vi "Read Variable_Values.vi"(8 "error in (no error)":errorcluster, 11 "muExpr in":refnum<class "mupExpr.lvclass">) -> (0 "error out":errorcluster, 2 "varValues":dbl[](array[numeric]), 3 "muExpr out":refnum<class "mupExpr.lvclass">)   [LabVIEW 2015, in "mupExpr.lvclass"]
uses:
  mupExpr.lvclass
  mupExpr.lvclass/mupExpr.ctl
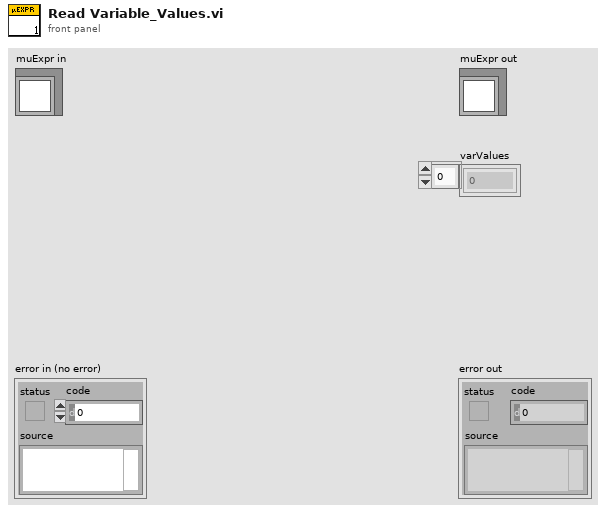
[diagram p1: front panel]
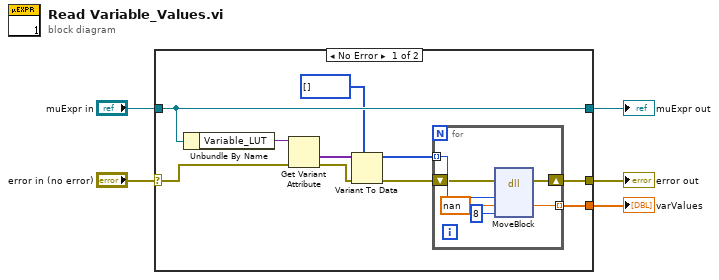
[diagram p0: block diagram]
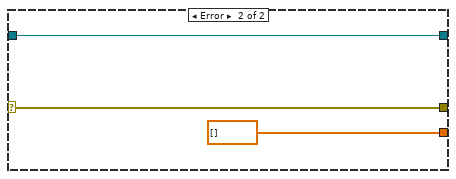
[diagram p2: hidden frame]
diagram:
  n1 = case shown="No Error" "error in (no error)" {
    selector: "error in (no error)" -> [w8 w24]
    tunnel: [w7 w24] -> w4
    tunnel: [w15 w23] -> w2
    tunnel: "muExpr in" -> [w15 w23]
    tunnel: [w6 dbl[] [] ("pd")] -> w1
    frame No Error {
      n2 = Unbundle By Name(w15) -> ("Variable_LUT"=w14:variant)
      n3 = Get Variant Attribute(Variant=w14, error in=w8) -> (values=w13:variant[], error out=w11:errorcluster)  [unwired: 2 in, 2 out]
      n4 = Variant To Data(error in=w11, type=u64[] [], Variant=w13) -> (data=w10:u64[], error out=w9:errorcluster)
      n5 = for {
        tunnel: w10 -> [w20] mode=indexing
        tunnel: [w17] -> w6 mode=indexing
        shift-right: [w16] -> w7
        shift-left: w9 -> [w19]
        n6 = dll-call lib="LabVIEW" fn="MoveBlock"(error in=w19, "ps"=w20, "pd"=nan, "size"=8) -> (error out=w16:errorcluster, "pd"=w17:dbl)  [unwired: 5 in, 1 out]
      }
    }
    frame Error {
    }
  }
  "error out" <- w4
  "muExpr out" <- w2
  "varValues" <- w1
